vi "Results_file_header.vi"() -> (0 "Header":string)   [LabVIEW 2010]
uses:
  Controls/Post_Process.ctl
  Globals/Meas_global.vi
panel:
  # "Create file Header"
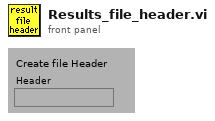
[diagram p1: front panel]
types:
  T1 = typedef "Post_Process.ctl" = enum16{"Take New Data", "Post Process Raw Data File"}
  T2 = typedef "Ch_and_Spans.ctl" = cluster{"high limit (10V)":sgl, "low limit (-10V)":sgl, "Ch No":i16, "Var name":string, "Use Latest Calib":bool}
  T3 = typedef "Board_Types.ctl" = enum16{"Simulate", "Local ADAM", "Server ADAM", "NI-DAQmx", "NI-DAQmxBase", "ADC488", "DT LV-link"}
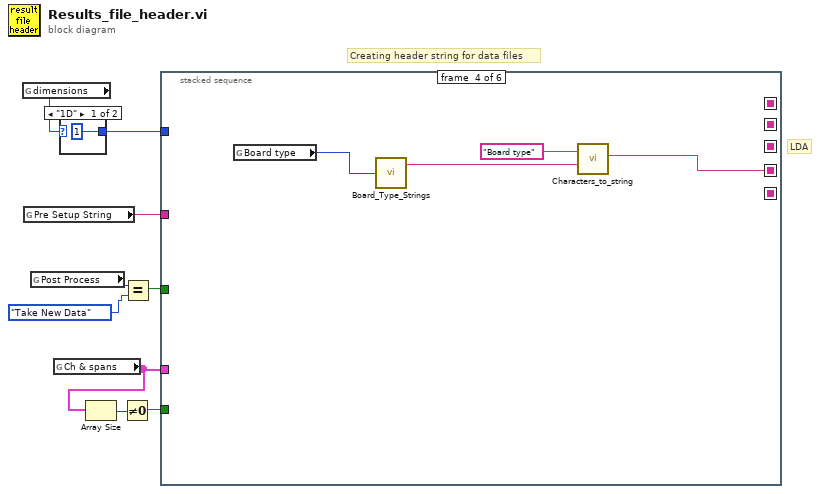
[diagram p0: block diagram]
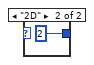
[diagram p2: hidden frame]
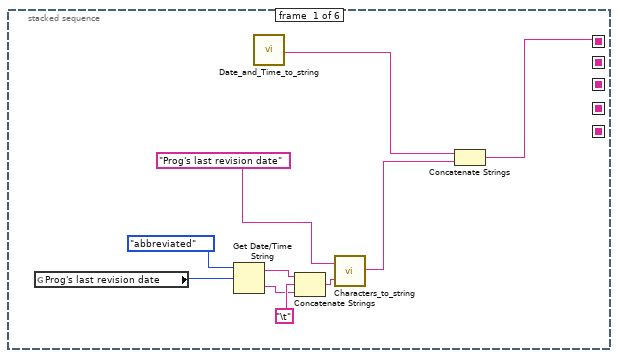
[diagram p3: hidden frame]
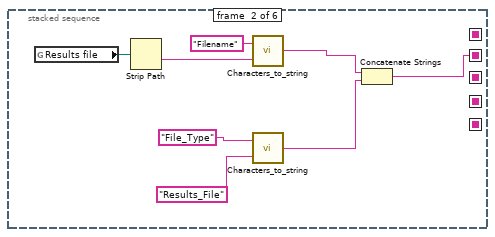
[diagram p4: hidden frame]
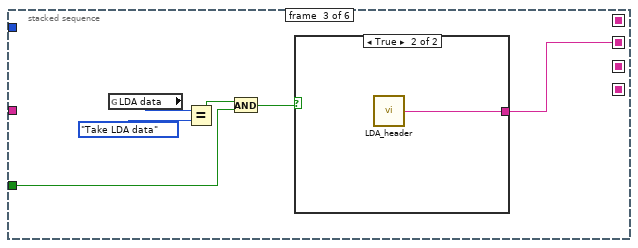
[diagram p5: hidden frame]
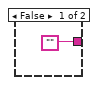
[diagram p6: hidden frame]
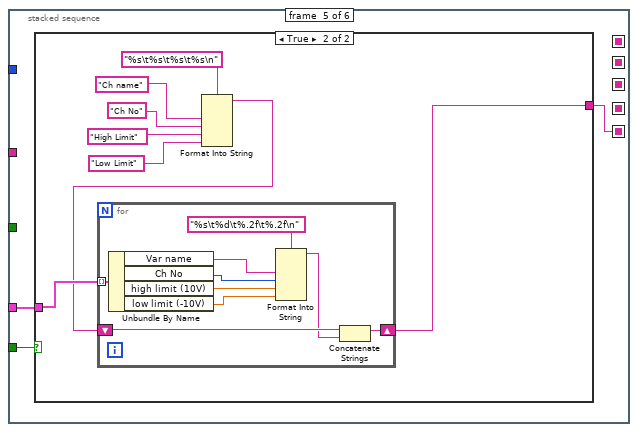
[diagram p7: hidden frame]
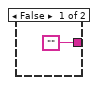
[diagram p8: hidden frame]
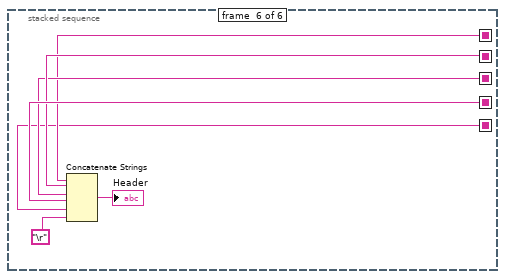
[diagram p9: hidden frame]
diagram:
  # "LDA"
  # "Creating header string for data files"
  n1 = global read "Meas_global.vi" "dimensions"() -> (w9:enum16{"1D", "2D"})
  n2 = global read "Meas_global.vi" "Pre Setup String"() -> (w2:string)
  n3 = global read "Meas_global.vi" "Post Process"() -> (w7:T1)
  n4 = global read "Meas_global.vi" "Ch & spans"() -> (w4:T2[])
  n5 = case shown="\"1D\"" w9 {
    tunnel: [1 2] -> w8
    frame "1D" {
    }
    frame "2D" {
    }
  }
  n6 = Array Size(array=w4) -> (size(s)=w5:i32)
  n7 = Not Equal To 0?(x=w5) -> (x != 0?=w3:bool)
  n8 = Equal?(x=w7, y=Post_Process."Take New Data" ("Post Process")) -> (x = y?=w6:bool)
  n9 = stacked-sequence {
    seq-local: [_ _ _ w38 _ _] -> [_ _ _ _ _ w69]
    seq-local: [_ w22 _ _ _ _] -> [_ _ _ _ _ w68]
    seq-local: [_ _ w31 _ _ _] -> [_ _ _ _ _ w67]
    seq-local: [w18 _ _ _ _ _] -> [_ _ _ _ _ w65]
    seq-local: [_ _ _ _ w42 _] -> [_ _ _ _ _ w64]
    tunnel: w8 -> [_ _ _ _ _ _]
    tunnel: w6 -> [_ _ w30 _ _ _]
    tunnel: w4 -> [_ _ _ _ w43 _]
    tunnel: w3 -> [_ _ _ _ w44 _]
    tunnel: w2 -> [_ _ _ _ _ _]
    frame #0 {
      n10 = global read "Meas_global.vi" "Prog's last revision date"() -> (w17:u32)
      n11 = Get Date/Time String(date format (0)=enum16{"short", "long", "abbreviated"}."abbreviated", seconds (now)=w17) -> (date string=w13:string, time string=w14:string)  [unwired: 1 out]
      n12 = call "Date_and_Time_to_string.vi"() -> ("Date and time (spreadsheet)"=w19:string)
      n13 = Concatenate Strings(w13, "\t", w14) -> (w12:string)
      n14 = call "Characters_to_string.vi"("Characters to write"=w12, "Label for characters"="Prog's last revision date") -> ("Output string"=w20:string)
      n15 = Concatenate Strings(w19, w20) -> (w18:string)
    }
    frame #1 {
      n16 = global read "Meas_global.vi" "Results file"() -> (w28:path)
      n17 = Strip Path(path=w28) -> (name=w27:string)  [unwired: 1 out]
      n18 = call "Characters_to_string.vi"("Characters to write"=w27, "Label for characters"="Filename") -> ("Output string"=w24:string)
      n19 = call "Characters_to_string.vi"("Characters to write"="Results_File", "Label for characters"="File_Type") -> ("Output string"=w23:string)
      n20 = Concatenate Strings(w24, w23) -> (w22:string)
    }
    frame #2 {
      n21 = global read "Meas_global.vi" "LDA data"() -> (w33:enum16{"No LDA data", "Take LDA data"})
      n22 = Equal?(x=w33, y=enum16{"No LDA data", "Take LDA data"}."Take LDA data" ("LDA data")) -> (x = y?=w35:bool)
      n23 = And(x=w35, y=w30) -> (x .and. y?=w32:bool)
      n24 = case shown="True" w32 {
        tunnel: ["" w37] -> w31
        frame False {
        }
        frame True {
          n25 = call "LDA_header.vi"() -> ("LDA Header string"=w37:string)  [unwired: 3 out]
        }
      }
    }
    frame #3 {
      n26 = global read "Meas_global.vi" "Board type"() -> (w39:T3)
      n27 = call "Board_Type_Strings.vi"("Board type"=w39) -> ("Board String"=w40:string)  [unwired: 1 out]
      n28 = call "Characters_to_string.vi"("Characters to write"=w40, "Label for characters"="Board type") -> ("Output string"=w38:string)
    }
    frame #4 {
      n29 = case shown="True" w44 {
        tunnel: w43 -> [_ w48]
        tunnel: ["" w46] -> w42
        frame False {
        }
        frame True {
          n30 = Format Into String(format string="%s\t%s\t%s\t%s\n" ("Format String"), "Ch name", "Ch No", "High Limit", "Low Limit") -> (resulting string=w47:string)  [unwired: 2 in, 1 out]
          n31 = for {
            tunnel: w48 -> [w62] mode=indexing
            shift-right: [w54] -> w46
            shift-left: w47 -> [w56]
            n32 = Unbundle By Name(w62) -> ("Var name"=w61:string, "Ch No"=w60:i16, "high limit (10V)"=w59:sgl, "low limit (-10V)"=w58:sgl)
            n33 = Format Into String(format string="%s\t%d\t%.2f\t%.2f\n" ("Format String"), w61, w60, w59, w58) -> (resulting string=w55:string)  [unwired: 2 in, 1 out]
            n34 = Concatenate Strings(w56, w55) -> (w54:string)
          }
        }
      }
    }
    frame #5 {
      n35 = Concatenate Strings(w65, w68, w67, w69, w64, "\r") -> (→"Header":string)
    }
  }
